vi "Update Progress.vi"(8 "error in (no error)":errorcluster, 9 "Current State":string, 10 "Test Name":string, 11 "User Interface in":refnum<class "User Interface.lvclass">) -> (0 "error out":errorcluster, 3 "User Interface out":refnum<class "User Interface.lvclass">)   [LabVIEW 2017, in "User Interface.lvlib" / "User Interface.lvclass"]
uses:
  User Interface.lvclass
  <vilib>/Utility/miscctls.llb/LVRowAndColumnTypeDef.ctl
  User Interface.lvclass/User Interface.ctl
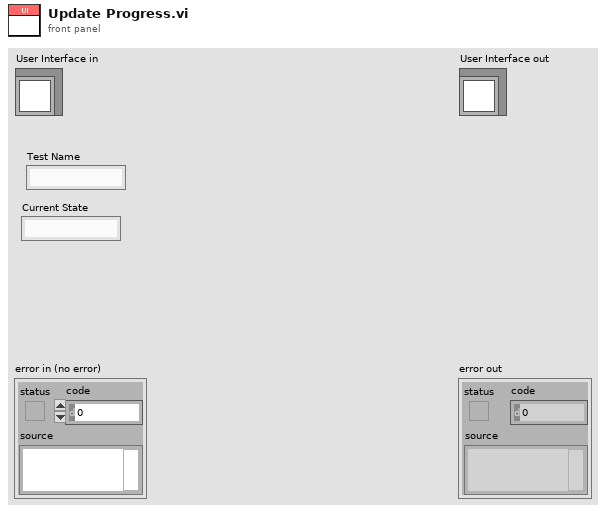
[diagram p1: front panel]
types:
  T1 = typedef "LVRowAndColumnTypeDef.ctl" = cluster{"Row":i32, "Column":i32}
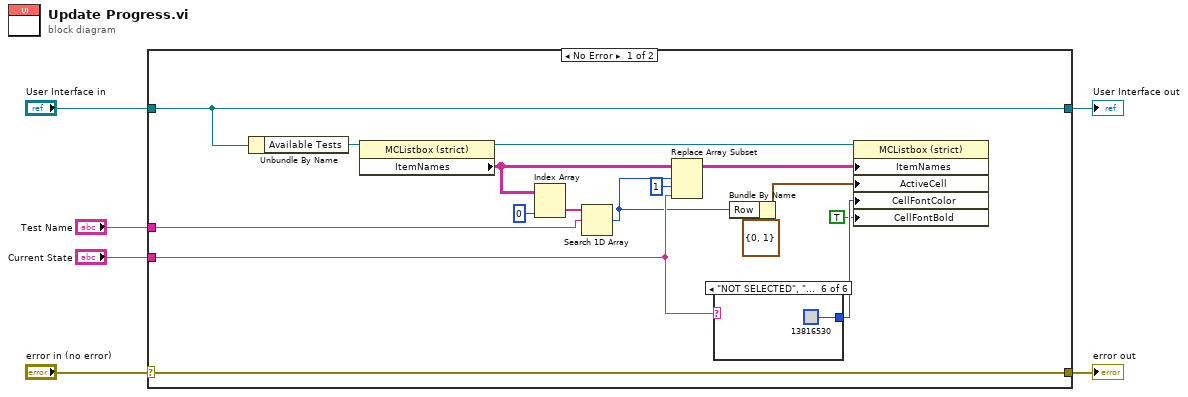
[diagram p0: block diagram]
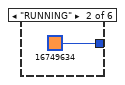
[diagram p3: hidden frame]
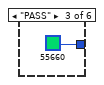
[diagram p4: hidden frame]
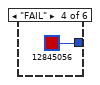
[diagram p5: hidden frame]
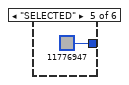
[diagram p6: hidden frame]
diagram:
  n1 = case shown="No Error" "error in (no error)" {
    selector: "error in (no error)" -> [w22 w29]
    tunnel: [w22 w29] -> w5
    tunnel: [w21 w28] -> w3
    tunnel: "User Interface in" -> [w21 w28]
    tunnel: "Current State" -> [w11 _]
    tunnel: "Test Name" -> [w17 _]
    frame No Error {
      n2 = Unbundle By Name(w21) -> ("Available Tests"=w20:refnum<vi>)
      n3 = property class="MCListbox (strict)"(reference=w20) -> (reference out=w13:refnum<vi>, "ItemNames"=w16:string[][])  [unwired: 1 in, 1 out]
      n4 = Index Array(array=w16, index (col)=0 ("disabled index (col)")) -> (element=w18:string[])  [unwired: 1 in]
      n5 = Search 1D Array(1D array=w18, element=w17) -> (index of element=w9:i32)  [unwired: 1 in]
      n6 = Replace Array Subset(array=w16, new element=w11, index (row)=w9, index (col)=1 ("disabled index (col)")) -> (w14:string[][])
      n7 = case shown="\"NOT SELECTED\", \"NOT STARTED\", \"SKIPPED\"" w11 {
        tunnel: [_ u32 16749634 ("Color Box") u32 55660 ("Color Box") u32 12845056 ("Color Box") u32 11776947 ("Color Box") u32 13816530 ("Color Box")] -> w8
        frame "False", Default {
        }
        frame "RUNNING" {
        }
        frame "PASS" {
        }
        frame "FAIL" {
        }
        frame "SELECTED" {
        }
        frame "NOT SELECTED", "NOT STARTED", "SKIPPED" {
        }
      }
      n8 = Bundle By Name(cluster=T1 {"Row"=0, "Column"=1} ("Active Cell:Active Cell"), "Row"=w9) -> (w10:T1)
      n9 = property class="MCListbox (strict)"(reference=w13, "ItemNames"=w14, "ActiveCell"=w10, "CellFontColor"=w8, "CellFontBold"=TRUE ("Active Cell:Cell Font:Bold")) -> ()  [unwired: 1 in, 2 out]
    }
    frame Error {
    }
  }
  "error out" <- w5
  "User Interface out" <- w3
